vi "Add New Menu Item Popup.vi"(8 "error in":errorcluster, 11 "Label In":string) -> (0 "error out":errorcluster, 2 "Path":string, 3 "Label Out":string)   [LabVIEW 2019]
doc: "All Rights Reserved © 2017 SyncSols"
uses:
  <vilib>/Utility/inputDevices.llb/keyboardAcquire.vi
panel:
  in  "Icon Path":path
  in  "Label Name":string
  # "<<Enter to Save the Changes>>"
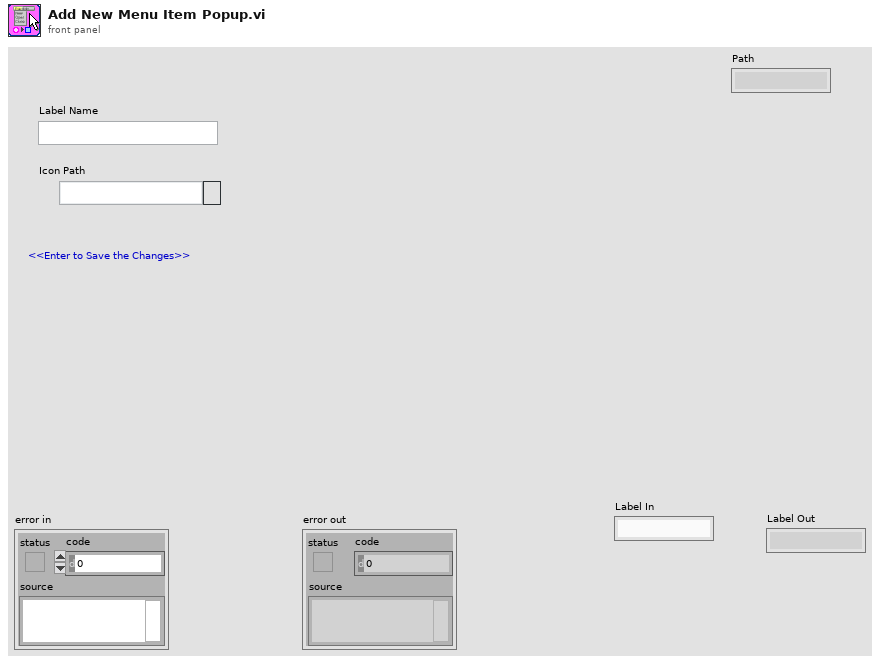
[diagram p1: front panel]
types:
  T1 = enum16{"0", "1", "2", "3", "4", "5", "6", "7", "8", "9", "A", "B", "C", "D", "E", "F", "G", "H", "I", "J", "K", "L", "M", "N", "O", "P", "Q", "R", "S", "T", "U", "V", "W", "X", "Y", "Z", "F1", "F2", "F3", "F4", "F5", "F6", "F7", "F8", "F9", "F10", "F11", "F12", "F13", "F14", "F15", "ADD", "BACK", "BACKSLASH", "CAPITAL", "COMMA", "DECIMAL", "DELETE", "DIVIDE", "DOWN", "END", "EQUALS", "ESCAPE", "GRAVE (`)", "HOME", "INSERT", "LBRACKET", "LCONTROL", "LEFT", "L ALT", "LSHIFT", "LWIN", "MINUS", "MULTIPLY", "NEXT", "NUMLOCK", "NUMPAD_0", "NUMPAD_1", "NUMPAD_2", "NUMPAD_3", "NUMPAD_4", "NUMPAD_5", "NUMPAD_6", "NUMPAD_7", "NUMPAD_8", "NUMPAD_9", "PAUSE", "PERIOD", "PRIOR (PG UP)", "RBRACKET", "RCONTROL", "RETURN", "RIGHT", "R ALT", "RSHIFT", "RWIN", "SCROLL", "SEMICOLON", "SLASH", "SPACE", "SUBTRACT", "TAB", "UP", "ENTER (num pad)", "' (quote)"}
  T2 = enum16{"0", "1", "2", "3", "4", "5", "6", "7", "8", "9", "A", "B", "C", "D", "E", "F", "G", "H", "I", "J", "K", "L", "M", "N", "O", "P", "Q", "R", "S", "T", "U", "V", "W", "X", "Y", "Z", "F1", "F2", "F3", "F4", "F5", "F6", "F7", "F8", "F9", "F10", "F11", "F12", "F13", "F14", "F15", "ADD", "BACK", "BACKSLASH", "CAPITAL", "COMMA", "DECIMAL", "DELETE", "DIVIDE", "DOWN", "END", "EQUALS", "ESCAPE", "GRAVE (`)", "HOME", "INSERT", "LBRACKET", "LCONTROL", "LEFT", "L ALT", "LSHIFT", "LWIN", "MINUS", "MULTIPLY", "NEXT", "NUMLOCK", "NUMPAD_0", "NUMPAD_1", "NUMPAD_2", "NUMPAD_3", "NUMPAD_4", "NUMPAD_5", "NUMPAD_6", "NUMPAD_7", "NUMPAD_8", "NUMPAD_9", "PAUSE", "PERIOD", "PRIOR (PG UP)", "RBRACKET", "RCONTROL", "RETURN", "RIGHT", "R ALT", "RSHIFT", "RWIN", "SCROLL", "SEMICOLON", "SLASH", "SPACE", "SUBTRACT", "TAB", "UP", "ENTER (num pad)", "' (quote)"}[]
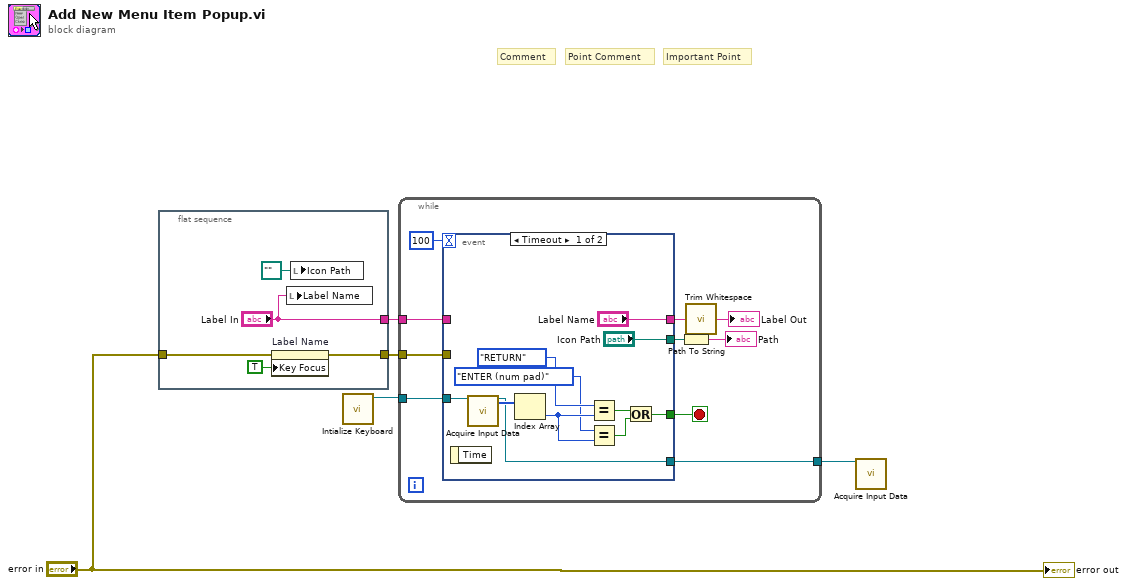
[diagram p0: block diagram]
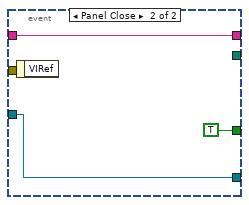
[diagram p2: hidden frame]
diagram:
  # "Important Point"
  # "Point Comment"
  # "Comment"
  n1 = flat-sequence {
    tunnel: "error in" -> [w9]
    tunnel: ["Label In"] -> w4
    tunnel: [w7] -> w1
    frame #0 {
      n2 = property on="Label Name" class="Str"(error in=w9, "Key Focus"=TRUE) -> (error out=w7:errorcluster)  [unwired: 1 in, 1 out]
      n3 = local write "Label Name"("Label In") -> ()
      n4 = local write "Icon Path"(path "" ("Icon Path")) -> ()
    }
  }
  n5 = call <vilib>:"Intialize Keyboard.vi"() -> ("device ID"=w3:refnum<k1>)  [unwired: 10 in, 1 out]
  n6 = while {
    tunnel: w4 -> [w17]
    tunnel: w3 -> [w16]
    tunnel: [w15] -> w2
    tunnel: w1 -> [w14]
    stop <- w18 stop-if-true
    n7 = event shown="[0] Timeout" {
      selector: _ -> [_ _]
      dyn-events: _ -> [_ _]
      timeout: 100 -> [_ _]
      tunnel: ["Label Name" w33] -> w20
      tunnel: [w25 TRUE] -> w18
      tunnel: w17 -> [_ w33]
      tunnel: w16 -> [w30 w32]
      tunnel: [w22 w32] -> w15
      tunnel: w14 -> [_ _]
      tunnel: ["Icon Path" _] -> w12
      event Timeout {
        n8 = event-data() -> ()  [unwired: 1 in, 1 out]
        n9 = call-poly <vilib>:"Acquire Input Data.vi"("device ID"=w30) -> ("device ID"=w22:refnum<k1>, "keys pressed"=w29:T2)  [unwired: 16 in, 1 out]
        n10 = Index Array(array=w29) -> (element=w27:T1)  [unwired: 1 in]
        n11 = Equal?(x=T1."RETURN" ("keyType 3"), y=w27) -> (x = y?=w24:bool)
        n12 = Equal?(x=T1."ENTER (num pad)" ("keyType 3"), y=w27) -> (x = y?=w23:bool)
        n13 = Or(x=w24, y=w23) -> (x .or. y?=w25:bool)
      }
      event Panel Close {
        n14 = event-data() -> ()  [unwired: 1 in, 1 out]
      }
    }
    n15 = Path To String(path=w12) -> (string=→"Path":string)
    n16 = call <vilib>:"Trim Whitespace.vi"("string"=w20) -> ("trimmed string"=→"Label Out":string)  [unwired: 1 in]
  }
  n17 = call-poly <vilib>:"Acquire Input Data.vi"("device ID"=w2) -> ()  [unwired: 16 in, 3 out]
  "error out" <- "error in"
